vi "recipeScript checkPythonCode.vi"(5 "userTable":string[][](array[string]), 6 "Python version(3.7.4)":string="3.7.4", 7 "instrTable":string[][](array[string]), 8 "error in (no error)":errorcluster, 10 "sourceFilePath":path, 11 "recipeScript":string) -> (0 "error out":errorcluster, 2 "scriptPythonCode":string, 3 "eventProcess":string[][](array[string]), 4 "showMsg":string[](array[string]))   [LabVIEW 2018]
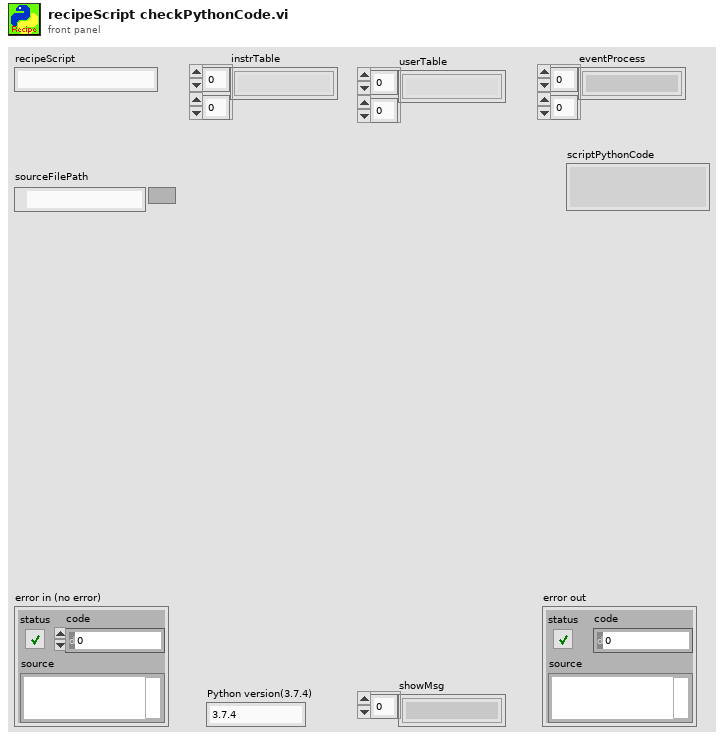
[diagram p1: front panel]
types:
  T1 = enum16{"open", "replace", "create", "open or create", "replace or create", "replace or create with confirmation"}
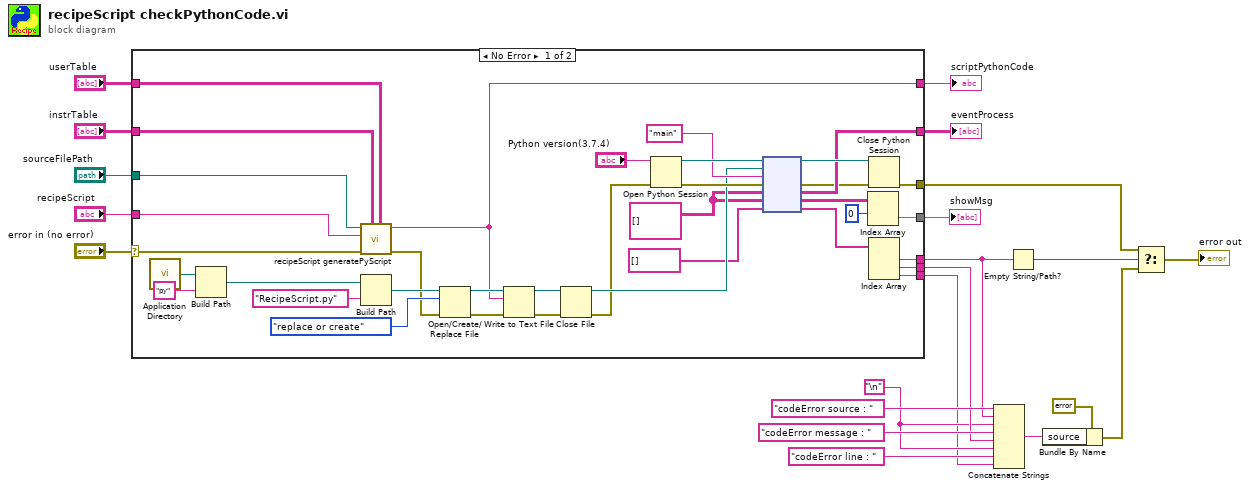
[diagram p0: block diagram]
diagram:
  w11 = "\n"
  n1 = case shown="No Error" "error in (no error)" {
    selector: "error in (no error)" -> [w26 w58]
    tunnel: "recipeScript" -> [w25 _]
    tunnel: [w41 _] -> w4
    tunnel: [w29 w58] -> w16
    tunnel: [w40 _] -> w14
    tunnel: [w39 _] -> w12
    tunnel: [w38 _] -> w9
    tunnel: "sourceFilePath" -> [w24 _]
    tunnel: [w23 _] -> w18
    tunnel: [w31 _] -> w5
    tunnel: "instrTable" -> [w28 _]
    tunnel: "userTable" -> [w27 _]
    frame No Error {
      w34 = string[][] []
      n2 = call <vilib>:"Application Directory.vi"() -> ("Application Directory"=w54:path)
      n3 = Build Path(base path=w54, name or relative path="py") -> (appended path=w56:path)
      n4 = call "recipeScript generatePyScript.vi"("userTable"=w27, "instrTable"=w28, "error in (no error)"=w26, "recipeScript"=w25, "sourceFilePath"=w24) -> ("error out"=w22:errorcluster, "PyCode"=w23:string)  [unwired: 5 in]
      n5 = Build Path(base path=w56, name or relative path="RecipeScript.py") -> (appended path=w49:path)
      n6 = Open/Create/Replace File(file path (use dialog)=w49, error in=w22, operation (0:open)=T1."replace or create") -> (refnum out=w53:refnum<file>, error out=w50:errorcluster)  [unwired: 3 in, 1 out]
      n7 = Write to Text File(file (use dialog)=w53, text=w23, error in=w50) -> (refnum out=w52:refnum<file>, error out=w51:errorcluster)  [unwired: 1 in, 1 out]
      n8 = Close File(refnum=w52, error in=w51) -> (path=w44:path, error out=w43:errorcluster)
      n9 = Open Python Session(python version="Python version(3.7.4)", 3:w43) -> (session out=w47:refnum<k35>, error out=w46:errorcluster)  [unwired: 1 in]
      n10 = node ("Python Node")(w47, w44, "main" ("function name"), w46, w34, w34, string[] []) -> (w42:refnum<k35>, w30:errorcluster, w41:string[][], w33:string[][], w36:string[])  [unwired: 2 out]
      n11 = Index Array(array=w33, index (row)=0) -> (element=w31:string[])  [unwired: 1 in]
      n12 = Close Python Session(session in=w42, error in=w30) -> (11:w29:errorcluster)
      n13 = Index Array(array=w36) -> (element #1=w40:string, element #2=w39:string, element #3=w38:string)  [unwired: 3 in]
    }
    frame Error {
    }
  }
  "eventProcess" <- w4
  "scriptPythonCode" <- w18
  "showMsg" <- w5
  n14 = Concatenate Strings("codeError source : ", w14, w11, "codeError message : ", w12, w11, "codeError line : ", w9) -> (w7:string)
  n15 = Empty String/Path?(string/path=w14) -> (empty?=w17:bool)
  n16 = Bundle By Name(cluster=errorcluster {"status"=TRUE, "code"=6999, "source"=""} ("f"), "source"=w7) -> (w6:errorcluster)
  n17 = Select(t=w16, s=w17, f=w6) -> (s? t:f=→"error out":errorcluster)
